vi "GetVisibillitySettings.vi"(0 "reference in":refnum<class "VINode.lvclass">, 5 "error in (no error)":errorcluster) -> (14 "reference out":refnum<class "VINode.lvclass">, 15 "showAttribute":bool, 16 "showMethods":bool, 19 "error out":errorcluster)   [LabVIEW 2020]
doc: "GetVisibillitySettings"
uses:
  <resource>/Framework/Providers/Open_GDS/UML/VINode_class/VINode.lvclass
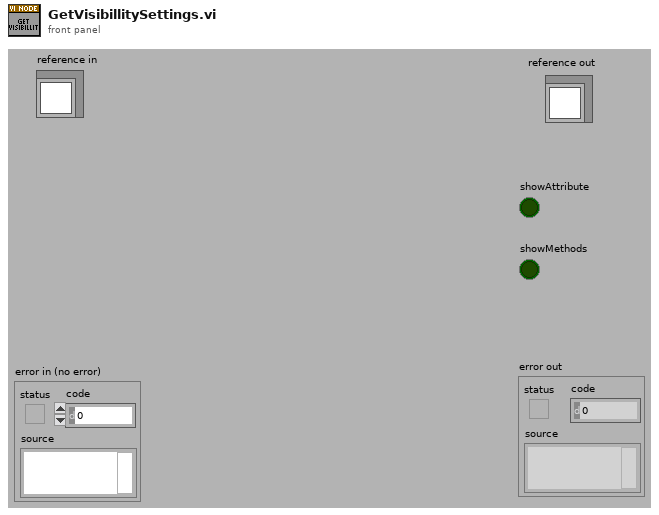
[diagram p1: front panel]
types:
  T1 = typedef "VINode.lvclass/ObjectAttributes.ctl" = cluster{"midHeight":dbl, "botHeight":dbl, "Name":refnum<class "MultiLineString.lvclass">, "DEFAULT_COMPARTMENT_HEIGHT":i32, "DEFAULT_WIDTH":i32, "DEFAULT_HEIGHT":i32, "VIPath":path, "Description":refnum<class "MultiLineString.lvclass">, "ShowDescription":bool}
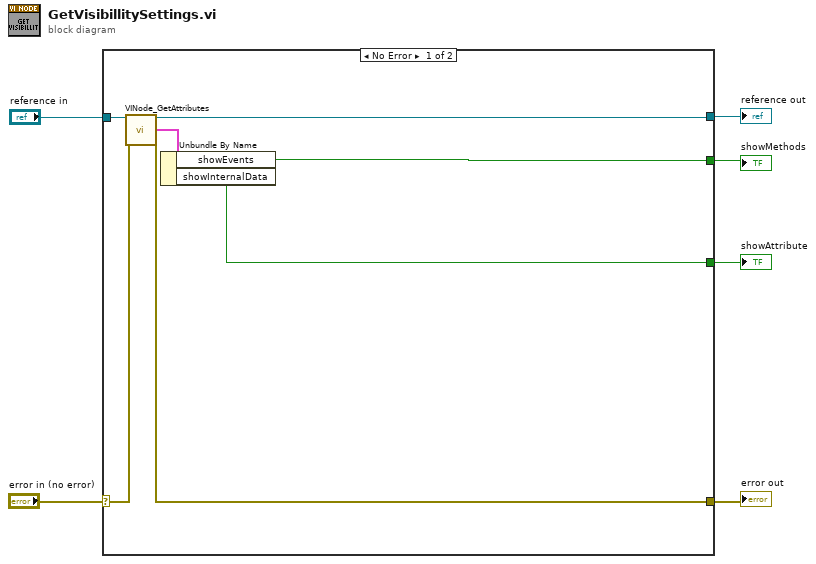
[diagram p0: block diagram]
diagram:
  n1 = case shown="No Error" "error in (no error)" {
    selector: "error in (no error)" -> [w13 w14]
    tunnel: "reference in" -> [w12 w15]
    tunnel: [w10 w14] -> w4
    tunnel: [w11 w15] -> w3
    tunnel: [w9 _] -> w2
    tunnel: [w8 _] -> w1
    frame No Error {
      n2 = call <resource>:"VINode_GetAttributes.vi"("reference in"=w12, "error in (no error)"=w13) -> ("reference out"=w11:refnum<class "VINode.lvclass">, "Data"=w7:T1, "error out"=w10:errorcluster)  [unwired: 1 in, 14 out]
      n3 = Unbundle By Name(w7) -> ("showEvents"=w9:bool, "showInternalData"=w8:bool)
    }
    frame Error {
    }
  }
  "reference out" <- w3
  "error out" <- w4
  "showMethods" <- w2
  "showAttribute" <- w1
